vi "BT 打印全流程2018-1.vi"(0 "文件路径":path, 1 "BT 具名数据源名称":string[](array[string]), 2 "输入内容":string[](array[string]), 3 "error in (no error)":errorcluster caption="错误输入（无错误）") -> (10 "error out":errorcluster caption="错误输出")   [LabVIEW 2018]
panel:
  in  "BarTender.IBtApplication":refnum<k7>
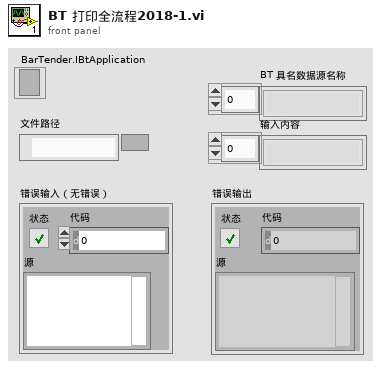
[diagram p1: front panel]
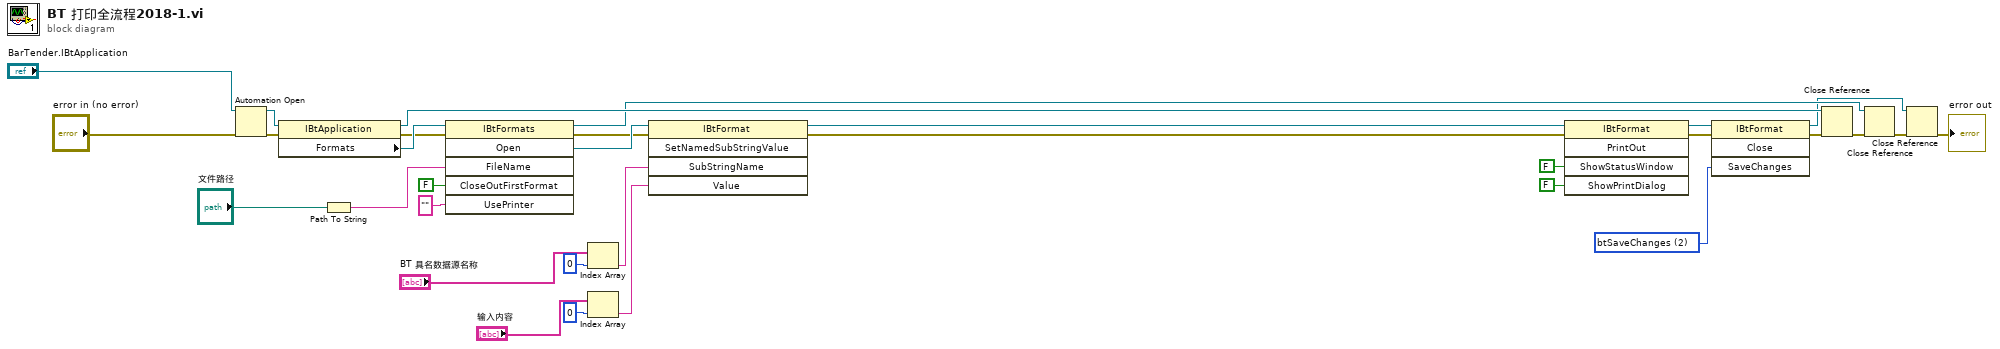
[diagram p0: block diagram]
diagram:
  w19 = 2 items=["btPromptSave", "btDoNotSaveChanges", "btSaveChanges"] ("SaveChanges")
  n1 = Automation Open(error in (no error)="error in (no error)", Automation Refnum="BarTender.IBtApplication") -> (Automation Refnum=w31:refnum<k7>, error out=w30:errorcluster)  [unwired: 2 in]
  n2 = property class="IBtApplication"(reference=w31, error in=w30) -> (reference out=w25:refnum<k7>, error out=w26:errorcluster, "Formats"=w29:refnum<k7>)
  n3 = Path To String(path="文件路径") -> (string=w21:string)
  n4 = invoke class="IBtFormats" method="Open"(reference=w29, error in=w26, "FileName"=w21, "CloseOutFirstFormat"=FALSE, "UsePrinter"="") -> (reference out=w24:refnum<k7>, error out=w9:errorcluster, "Open"=w10:refnum<k7>)  [unwired: 1 in, 3 out]
  n5 = Index Array(array="BT 具名数据源名称", index=0) -> (element=w7:string)
  n6 = Index Array(array="输入内容", index=0) -> (element=w6:string)
  n7 = invoke class="IBtFormat" method="SetNamedSubStringValue"(reference=w10, error in=w9, "SubStringName"=w7, "Value"=w6) -> (reference out=w2:refnum<k7>, error out=w1:errorcluster)  [unwired: 1 in, 3 out]
  n8 = invoke class="IBtFormat" method="PrintOut"(reference=w2, error in=w1, "ShowStatusWindow"=FALSE, "ShowPrintDialog"=FALSE) -> (reference out=w12:refnum<k7>, error out=w11:errorcluster)  [unwired: 1 in, 3 out]
  n9 = invoke class="IBtFormat" method="Close"(reference=w12, error in=w11, "SaveChanges"=w19) -> (reference out=w18:refnum<k7>, error out=w17:errorcluster)  [unwired: 1 in, 2 out]
  n10 = Close Reference(reference=w25, error in (no error)=w17) -> (error out=w23:errorcluster)
  n11 = Close Reference(reference=w24, error in (no error)=w23) -> (error out=w16:errorcluster)
  n12 = Close Reference(reference=w18, error in (no error)=w16) -> (error out=→"error out":errorcluster)
